vi "HDF5_Write_Disdrometer_Record.vi"(0 "DisdromRefs":T4 {"Status_dset_deprecated" format="%.0x"; "Spectrum_dset" format="%.0x"; "SpectGroup_ref" format="%.0x"; "HydromType_dset" format="%.0x"; "UnknownVolum_dset" format="%.0x"; "UnknownParticls_dset" format="%.0x"; "NonHydrVolum_dset" format="%.0x"; "NonHydrParticls_dset" format="%.0x"; "ParticlMinDiam_dset" format="%.0x"; "ParticlMaxSpeed_dset" format="%.0x"; "RadarReflect_dset" format="%.0x"; "Visibility_dset" format="%.0x"; "TotalRain_dset" format="%.0x"; "Solid_dset" format="%.0x"; "Liquid_dset" format="%.0x"; "TotalRainRate_dset" format="%.0x"; "TimeStamp_dset" format="%.0x"; "ParticlMinSpeed_dset" format="%.0x"; "MeasdParticles_dset" format="%.0x"; "MaxDiam_dset" format="%.0x"; "BasicGroup_ref" format="%.0x"}, 7 "DisdrometerData":T1={"Spectrum Data"=[], "DisdromSummary"={"current time"=0.0, "Timestamp"=0.0, "Total Rain Rate"=0.0, "Liquid Rain Rate"=0.0, "Solid Rain Rate"=0.0, "Total Rainfall"=0.0, "Visibility"=0.0, "Radar Reflectivity"=0.0, "Max Diameter Hail"=0.0, "Measured Particles"=0, "Particle Min Speed"=0, "Particle Max Speed"=0, "Particle Min Diam"=0, "NonHydr Particles"=0, "NonHydr Volume"=0.0, "Unkn Particles"=0, "Unkn Volume"=0.0, "HydroType"=0}, "Status"={"Laser"=TRUE, "Signal"=TRUE, "LaserTemp_Analog"=TRUE, "LaserTemp_Digital"=TRUE, "LaserCurrent_Analog"=TRUE, "LaserCurrent_Digital"=TRUE, "SensorSupply"=TRUE, "HeatLaserHead"=TRUE, "HeatReceiverHead"=TRUE, "TempSensor"=TRUE, "HeatSupply"=TRUE, "HeatHousing"=TRUE, "HeatHeads"=TRUE, "HeatCarriers"=TRUE, "OutputLaserPower"=TRUE, "Checksum"=TRUE, "StatusInt"=0}}, 11 "error in":errorcluster) -> (15 "error out":errorcluster)   [LabVIEW 2018]
doc: "Write a single Noise<x> record with timestamp:\nNoise1\n NoiseInfo - cluster with Timestamp and other metadata for this record\n SummdSpectrum - 1024 element Double array (waveform)"
uses:
  HDF5_Disdrometer_Refs.ctl
  <vilib>/addons/h5labview2/base/hid_t.ctl
  DisdrometerData.ctl
  DisdromterSummaryData.ctl
  Disdrometer/Disdrometer_Status_Cluster.ctl
  lib_path_mod_20200519.vi
  <vilib>/addons/h5labview2/base/H5Equery.vi
  <vilib>/addons/h5labview2/base/lib_path.vi
  <vilib>/addons/h5labview2/dataset/H5Dwrite.llb/H5Dwrite.xnode
  <vilib>/addons/h5labview2/dataset/H5D.lvlib
  <vilib>/addons/h5labview2/space/H5S.lvlib
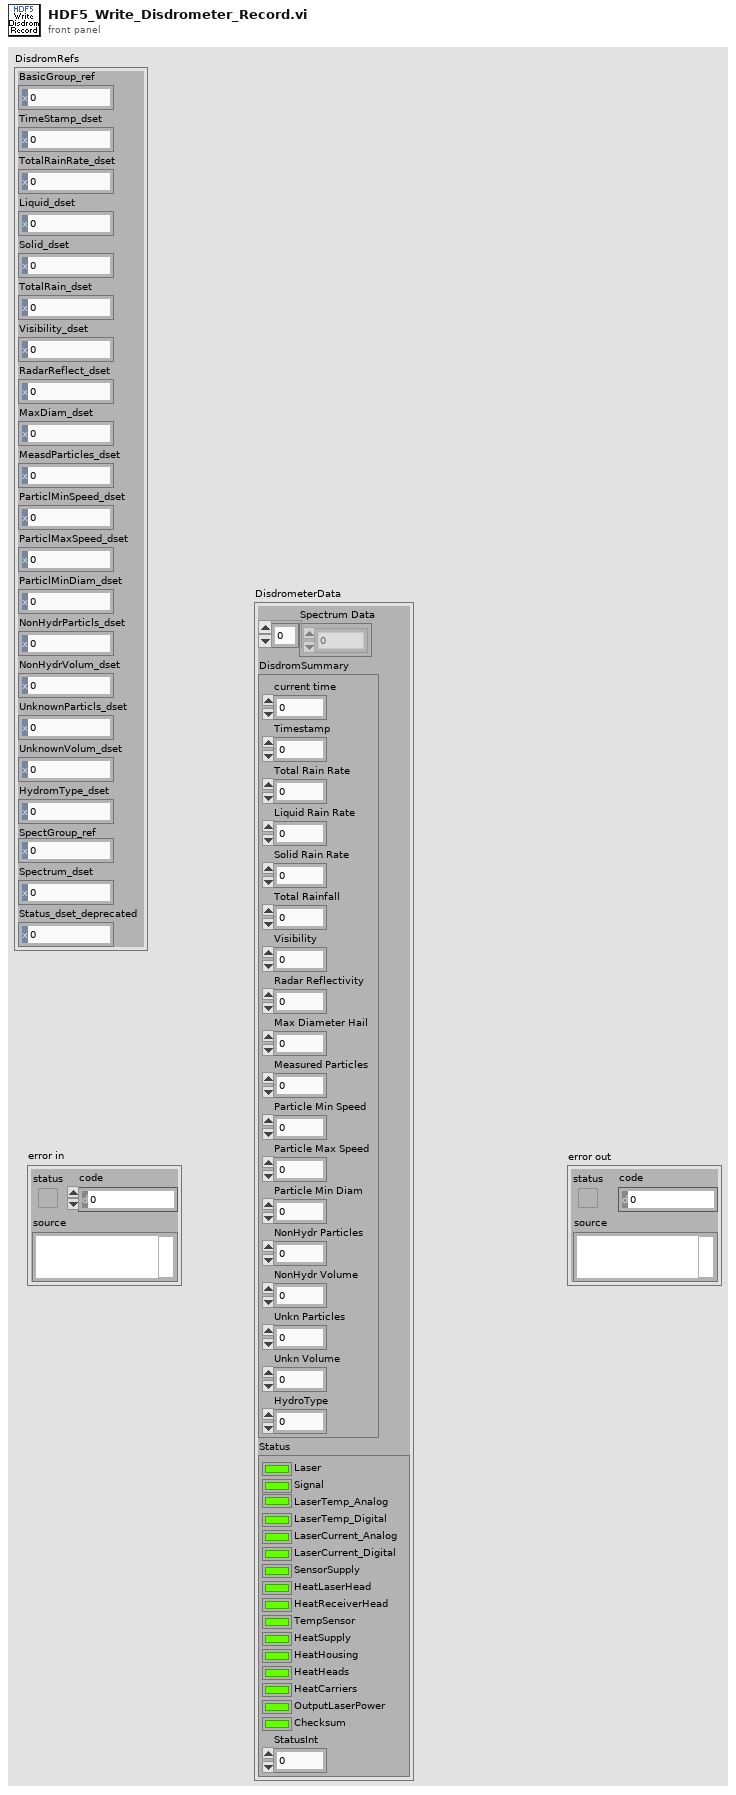
[diagram p1: front panel]
types:
  T1 = typedef "DisdrometerData.ctl" = cluster{"Spectrum Data":i16[], "DisdromSummary":T2, "Status":T3}
  T2 = typedef "DisdromterSummaryData.ctl" = cluster{"current time":dbl, "Timestamp":dbl, "Total Rain Rate":dbl, "Liquid Rain Rate":dbl, "Solid Rain Rate":dbl, "Total Rainfall":dbl, "Visibility":dbl, "Radar Reflectivity":dbl, "Max Diameter Hail":dbl, "Measured Particles":i32, "Particle Min Speed":i16, "Particle Max Speed":i16, "Particle Min Diam":i16, "NonHydr Particles":i16, "NonHydr Volume":dbl, "Unkn Particles":i16, "Unkn Volume":dbl, "HydroType":i8}
  T3 = typedef "Disdrometer_Status_Cluster.ctl" = cluster{"Laser":bool, "Signal":bool, "LaserTemp_Analog":bool, "LaserTemp_Digital":bool, "LaserCurrent_Analog":bool, "LaserCurrent_Digital":bool, "SensorSupply":bool, "HeatLaserHead":bool, "HeatReceiverHead":bool, "TempSensor":bool, "HeatSupply":bool, "HeatHousing":bool, "HeatHeads":bool, "HeatCarriers":bool, "OutputLaserPower":bool, "Checksum":bool, "StatusInt":u16}
  T4 = typedef "HDF5_Disdrometer_Refs.ctl" = cluster{"BasicGroup_ref":T5, "TimeStamp_dset":T5, "TotalRainRate_dset":T5, "Liquid_dset":T5, "Solid_dset":T5, "TotalRain_dset":T5, "Visibility_dset":T5, "RadarReflect_dset":T5, "MaxDiam_dset":T5, "MeasdParticles_dset":T5, "ParticlMinSpeed_dset":T5, "ParticlMaxSpeed_dset":T5, "ParticlMinDiam_dset":T5, "NonHydrParticls_dset":T5, "NonHydrVolum_dset":T5, "UnknownParticls_dset":T5, "UnknownVolum_dset":T5, "HydromType_dset":T5, "SpectGroup_ref":T5, "Spectrum_dset":T5, "Status_dset_deprecated":T5}
  T5 = typedef "hid_t.ctl" = i32
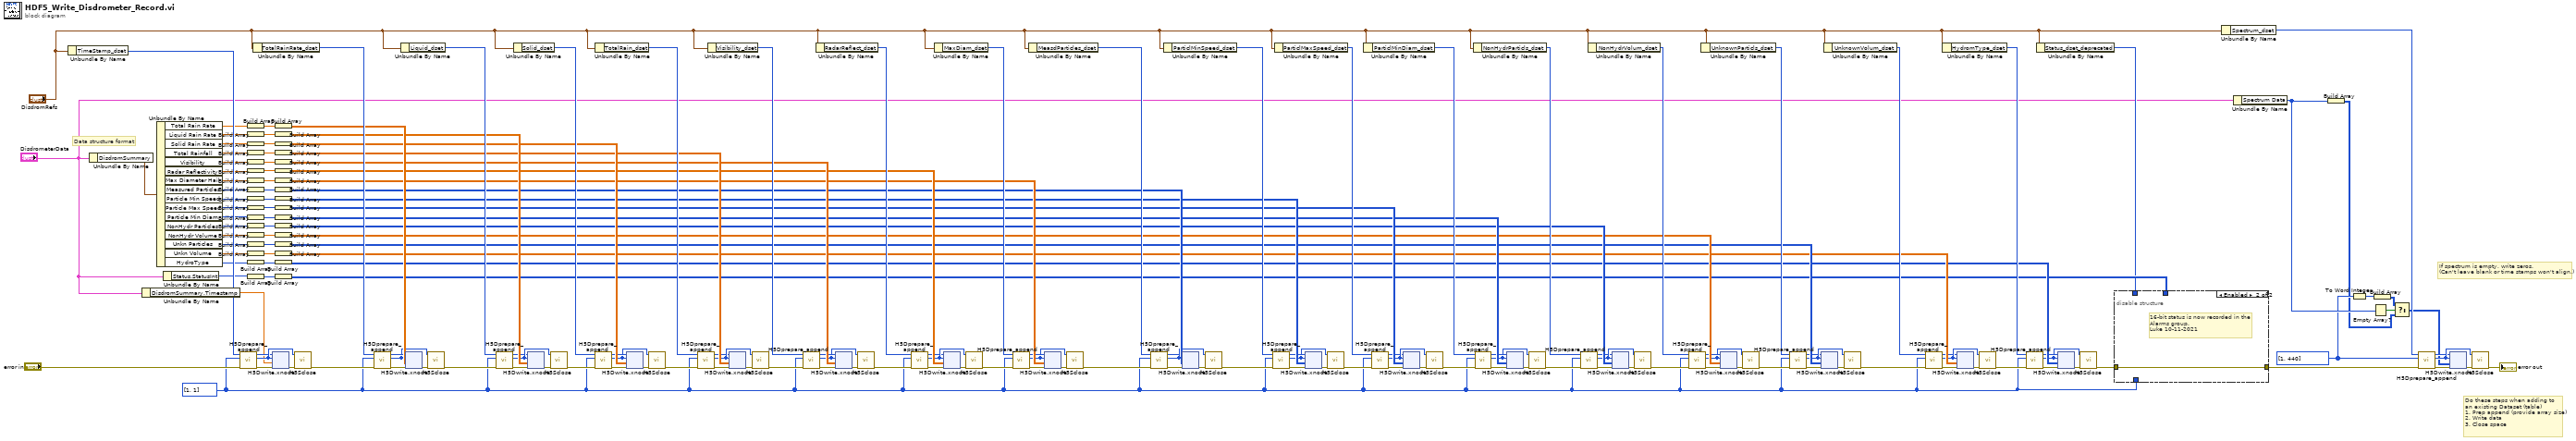
[diagram p0: block diagram]
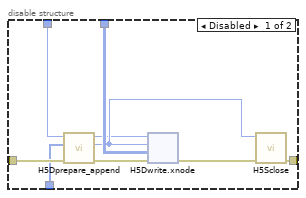
[diagram p2: hidden frame]
diagram:
  w6 = u64[] [1, 440] ("append dims")
  w17 = i32[] [1, 1] ("size(s)")
  # "If spectrum is empty, write zeros.\n(Can't leave blank or time stamps won't align.)"
  # "Data structure format"
  # "Do these steps when adding to \nan existing Dataset (table)\n1. Prep append (provide array size)\n2. Write data\n3. Close space"
  n1 = Unbundle By Name("DisdromRefs") -> ("TimeStamp_dset"=w174:T5)
  n2 = Unbundle By Name("DisdrometerData") -> ("DisdromSummary"=w132:T2)
  n3 = Unbundle By Name("DisdrometerData") -> ("DisdromSummary.Timestamp"=w1:dbl)
  n4 = Unbundle By Name(w132) -> ("Total Rain Rate"=w99:dbl, "Liquid Rain Rate"=w22:dbl, "Solid Rain Rate"=w23:dbl, "Total Rainfall"=w24:dbl, "Visibility"=w25:dbl, "Radar Reflectivity"=w26:dbl, "Max Diameter Hail"=w27:dbl, "Measured Particles"=w28:i32, "Particle Min Speed"=w29:i16, "Particle Max Speed"=w30:i16, "Particle Min Diam"=w31:i16, "NonHydr Particles"=w32:i16, "NonHydr Volume"=w33:dbl, "Unkn Particles"=w34:i16, "Unkn Volume"=w35:dbl, "HydroType"=w36:i8)
  n5 = Unbundle By Name("DisdrometerData") -> ("Status.StatusInt"=w21:u16)
  n6 = call <vilib>:"H5Dprepare_append.vi"("error in (no error)"="error in", "append dims"=w17, "dset in"=w174) -> ("error out"=w136:errorcluster, "space out"=w134:T5, "dset out"=w133:T5)  [unwired: 5 in, 1 out]
  n7 = Build Array(w99) -> (w52:dbl[])
  n8 = Build Array(w22) -> (w51:dbl[])
  n9 = Build Array(w23) -> (w49:dbl[])
  n10 = Build Array(w24) -> (w50:dbl[])
  n11 = Build Array(w25) -> (w45:dbl[])
  n12 = Build Array(w26) -> (w46:dbl[])
  n13 = Build Array(w27) -> (w48:dbl[])
  n14 = Build Array(w28) -> (w47:i32[])
  n15 = Build Array(w29) -> (w37:i16[])
  n16 = Build Array(w30) -> (w38:i16[])
  n17 = Build Array(w31) -> (w40:i16[])
  n18 = Build Array(w32) -> (w39:i16[])
  n19 = Build Array(w33) -> (w44:dbl[])
  n20 = Build Array(w34) -> (w43:i16[])
  n21 = Build Array(w35) -> (w41:dbl[])
  n22 = Build Array(w36) -> (w42:i8[])
  n23 = Build Array(w21) -> (w20:u16[])
  n24 = Unbundle By Name("DisdromRefs") -> ("TotalRainRate_dset"=w172:T5)
  n25 = xnode "H5Dwrite.xnode"("error in (no error)"=w136, "data"=w1, "file space"=w134, "ref in"=w133) -> ("error out"=w135:errorcluster)  [unwired: 3 in, 2 out]
  n26 = Build Array(w52) -> (w156:dbl[][])
  n27 = Build Array(w51) -> (w155:dbl[][])
  n28 = Build Array(w49) -> (w154:dbl[][])
  n29 = Build Array(w50) -> (w153:dbl[][])
  n30 = Build Array(w45) -> (w152:dbl[][])
  n31 = Build Array(w46) -> (w151:dbl[][])
  n32 = Build Array(w48) -> (w150:dbl[][])
  n33 = Build Array(w47) -> (w149:i32[][])
  n34 = Build Array(w37) -> (w148:i16[][])
  n35 = Build Array(w38) -> (w147:i16[][])
  n36 = Build Array(w40) -> (w146:i16[][])
  n37 = Build Array(w39) -> (w145:i16[][])
  n38 = Build Array(w44) -> (w144:dbl[][])
  n39 = Build Array(w43) -> (w143:i16[][])
  n40 = Build Array(w41) -> (w142:dbl[][])
  n41 = Build Array(w42) -> (w141:i8[][])
  n42 = Build Array(w20) -> (w16:u16[][])
  n43 = call <vilib>:"H5Sclose.vi"("error in (no error)"=w135, "space in"=w134) -> ("error out"=w118:errorcluster)  [unwired: 9 in]
  n44 = call <vilib>:"H5Dprepare_append.vi"("error in (no error)"=w118, "append dims"=w17, "dset in"=w172) -> ("error out"=w137:errorcluster, "space out"=w139:T5, "dset out"=w140:T5)  [unwired: 5 in, 1 out]
  n45 = Unbundle By Name("DisdromRefs") -> ("Liquid_dset"=w171:T5)
  n46 = xnode "H5Dwrite.xnode"("error in (no error)"=w137, "data"=w156, "file space"=w139, "ref in"=w140) -> ("error out"=w138:errorcluster)  [unwired: 3 in, 2 out]
  n47 = call <vilib>:"H5Sclose.vi"("error in (no error)"=w138, "space in"=w139) -> ("error out"=w117:errorcluster)  [unwired: 9 in]
  n48 = call <vilib>:"H5Dprepare_append.vi"("error in (no error)"=w117, "append dims"=w17, "dset in"=w171) -> ("error out"=w131:errorcluster, "space out"=w129:T5, "dset out"=w128:T5)  [unwired: 5 in, 1 out]
  n49 = Unbundle By Name("DisdromRefs") -> ("Solid_dset"=w170:T5)
  n50 = xnode "H5Dwrite.xnode"("error in (no error)"=w131, "data"=w155, "file space"=w129, "ref in"=w128) -> ("error out"=w130:errorcluster)  [unwired: 3 in, 2 out]
  n51 = call <vilib>:"H5Sclose.vi"("error in (no error)"=w130, "space in"=w129) -> ("error out"=w116:errorcluster)  [unwired: 9 in]
  n52 = call <vilib>:"H5Dprepare_append.vi"("error in (no error)"=w116, "append dims"=w17, "dset in"=w170) -> ("error out"=w124:errorcluster, "space out"=w126:T5, "dset out"=w127:T5)  [unwired: 5 in, 1 out]
  n53 = Unbundle By Name("DisdromRefs") -> ("TotalRain_dset"=w169:T5)
  n54 = xnode "H5Dwrite.xnode"("error in (no error)"=w124, "data"=w154, "file space"=w126, "ref in"=w127) -> ("error out"=w125:errorcluster)  [unwired: 3 in, 2 out]
  n55 = call <vilib>:"H5Sclose.vi"("error in (no error)"=w125, "space in"=w126) -> ("error out"=w115:errorcluster)  [unwired: 9 in]
  n56 = call <vilib>:"H5Dprepare_append.vi"("error in (no error)"=w115, "append dims"=w17, "dset in"=w169) -> ("error out"=w123:errorcluster, "space out"=w121:T5, "dset out"=w120:T5)  [unwired: 5 in, 1 out]
  n57 = Unbundle By Name("DisdromRefs") -> ("Visibility_dset"=w168:T5)
  n58 = xnode "H5Dwrite.xnode"("error in (no error)"=w123, "data"=w153, "file space"=w121, "ref in"=w120) -> ("error out"=w122:errorcluster)  [unwired: 3 in, 2 out]
  n59 = call <vilib>:"H5Sclose.vi"("error in (no error)"=w122, "space in"=w121) -> ("error out"=w110:errorcluster)  [unwired: 9 in]
  n60 = call <vilib>:"H5Dprepare_append.vi"("error in (no error)"=w110, "append dims"=w17, "dset in"=w168) -> ("error out"=w111:errorcluster, "space out"=w113:T5, "dset out"=w114:T5)  [unwired: 5 in, 1 out]
  n61 = Unbundle By Name("DisdromRefs") -> ("RadarReflect_dset"=w167:T5)
  n62 = xnode "H5Dwrite.xnode"("error in (no error)"=w111, "data"=w152, "file space"=w113, "ref in"=w114) -> ("error out"=w112:errorcluster)  [unwired: 3 in, 2 out]
  n63 = call <vilib>:"H5Sclose.vi"("error in (no error)"=w112, "space in"=w113) -> ("error out"=w105:errorcluster)  [unwired: 9 in]
  n64 = call <vilib>:"H5Dprepare_append.vi"("error in (no error)"=w105, "append dims"=w17, "dset in"=w167) -> ("error out"=w109:errorcluster, "space out"=w107:T5, "dset out"=w106:T5)  [unwired: 5 in, 1 out]
  n65 = Unbundle By Name("DisdromRefs") -> ("MaxDiam_dset"=w166:T5)
  n66 = xnode "H5Dwrite.xnode"("error in (no error)"=w109, "data"=w151, "file space"=w107, "ref in"=w106) -> ("error out"=w108:errorcluster)  [unwired: 3 in, 2 out]
  n67 = call <vilib>:"H5Sclose.vi"("error in (no error)"=w108, "space in"=w107) -> ("error out"=w100:errorcluster)  [unwired: 9 in]
  n68 = call <vilib>:"H5Dprepare_append.vi"("error in (no error)"=w100, "append dims"=w17, "dset in"=w166) -> ("error out"=w101:errorcluster, "space out"=w103:T5, "dset out"=w104:T5)  [unwired: 5 in, 1 out]
  n69 = Unbundle By Name("DisdromRefs") -> ("MeasdParticles_dset"=w159:T5)
  n70 = xnode "H5Dwrite.xnode"("error in (no error)"=w101, "data"=w150, "file space"=w103, "ref in"=w104) -> ("error out"=w102:errorcluster)  [unwired: 3 in, 2 out]
  n71 = call <vilib>:"H5Sclose.vi"("error in (no error)"=w102, "space in"=w103) -> ("error out"=w64:errorcluster)  [unwired: 9 in]
  n72 = call <vilib>:"H5Dprepare_append.vi"("error in (no error)"=w64, "append dims"=w17, "dset in"=w159) -> ("error out"=w68:errorcluster, "space out"=w66:T5, "dset out"=w65:T5)  [unwired: 5 in, 1 out]
  n73 = Unbundle By Name("DisdromRefs") -> ("ParticlMinSpeed_dset"=w160:T5)
  n74 = xnode "H5Dwrite.xnode"("error in (no error)"=w68, "data"=w149, "file space"=w66, "ref in"=w65) -> ("error out"=w67:errorcluster)  [unwired: 3 in, 2 out]
  n75 = call <vilib>:"H5Sclose.vi"("error in (no error)"=w67, "space in"=w66) -> ("error out"=w81:errorcluster)  [unwired: 9 in]
  n76 = call <vilib>:"H5Dprepare_append.vi"("error in (no error)"=w81, "append dims"=w17, "dset in"=w160) -> ("error out"=w69:errorcluster, "space out"=w71:T5, "dset out"=w72:T5)  [unwired: 5 in, 1 out]
  n77 = Unbundle By Name("DisdromRefs") -> ("ParticlMaxSpeed_dset"=w161:T5)
  n78 = xnode "H5Dwrite.xnode"("error in (no error)"=w69, "data"=w148, "file space"=w71, "ref in"=w72) -> ("error out"=w70:errorcluster)  [unwired: 3 in, 2 out]
  n79 = call <vilib>:"H5Sclose.vi"("error in (no error)"=w70, "space in"=w71) -> ("error out"=w82:errorcluster)  [unwired: 9 in]
  n80 = Unbundle By Name("DisdromRefs") -> ("ParticlMinDiam_dset"=w162:T5)
  n81 = call <vilib>:"H5Dprepare_append.vi"("error in (no error)"=w82, "append dims"=w17, "dset in"=w161) -> ("error out"=w76:errorcluster, "space out"=w74:T5, "dset out"=w73:T5)  [unwired: 5 in, 1 out]
  n82 = xnode "H5Dwrite.xnode"("error in (no error)"=w76, "data"=w147, "file space"=w74, "ref in"=w73) -> ("error out"=w75:errorcluster)  [unwired: 3 in, 2 out]
  n83 = call <vilib>:"H5Sclose.vi"("error in (no error)"=w75, "space in"=w74) -> ("error out"=w83:errorcluster)  [unwired: 9 in]
  n84 = Unbundle By Name("DisdromRefs") -> ("NonHydrParticls_dset"=w163:T5)
  n85 = call <vilib>:"H5Dprepare_append.vi"("error in (no error)"=w83, "append dims"=w17, "dset in"=w162) -> ("error out"=w77:errorcluster, "space out"=w79:T5, "dset out"=w80:T5)  [unwired: 5 in, 1 out]
  n86 = xnode "H5Dwrite.xnode"("error in (no error)"=w77, "data"=w146, "file space"=w79, "ref in"=w80) -> ("error out"=w78:errorcluster)  [unwired: 3 in, 2 out]
  n87 = call <vilib>:"H5Sclose.vi"("error in (no error)"=w78, "space in"=w79) -> ("error out"=w88:errorcluster)  [unwired: 9 in]
  n88 = call <vilib>:"H5Dprepare_append.vi"("error in (no error)"=w88, "append dims"=w17, "dset in"=w163) -> ("error out"=w87:errorcluster, "space out"=w85:T5, "dset out"=w84:T5)  [unwired: 5 in, 1 out]
  n89 = Unbundle By Name("DisdromRefs") -> ("NonHydrVolum_dset"=w164:T5)
  n90 = xnode "H5Dwrite.xnode"("error in (no error)"=w87, "data"=w145, "file space"=w85, "ref in"=w84) -> ("error out"=w86:errorcluster)  [unwired: 3 in, 2 out]
  n91 = call <vilib>:"H5Sclose.vi"("error in (no error)"=w86, "space in"=w85) -> ("error out"=w93:errorcluster)  [unwired: 9 in]
  n92 = call <vilib>:"H5Dprepare_append.vi"("error in (no error)"=w93, "append dims"=w17, "dset in"=w164) -> ("error out"=w89:errorcluster, "space out"=w91:T5, "dset out"=w92:T5)  [unwired: 5 in, 1 out]
  n93 = Unbundle By Name("DisdromRefs") -> ("UnknownParticls_dset"=w165:T5)
  n94 = xnode "H5Dwrite.xnode"("error in (no error)"=w89, "data"=w144, "file space"=w91, "ref in"=w92) -> ("error out"=w90:errorcluster)  [unwired: 3 in, 2 out]
  n95 = call <vilib>:"H5Sclose.vi"("error in (no error)"=w90, "space in"=w91) -> ("error out"=w98:errorcluster)  [unwired: 9 in]
  n96 = call <vilib>:"H5Dprepare_append.vi"("error in (no error)"=w98, "append dims"=w17, "dset in"=w165) -> ("error out"=w97:errorcluster, "space out"=w95:T5, "dset out"=w94:T5)  [unwired: 5 in, 1 out]
  n97 = xnode "H5Dwrite.xnode"("error in (no error)"=w97, "data"=w143, "file space"=w95, "ref in"=w94) -> ("error out"=w96:errorcluster)  [unwired: 3 in, 2 out]
  n98 = Unbundle By Name("DisdromRefs") -> ("UnknownVolum_dset"=w158:T5)
  n99 = call <vilib>:"H5Sclose.vi"("error in (no error)"=w96, "space in"=w95) -> ("error out"=w54:errorcluster)  [unwired: 9 in]
  n100 = call <vilib>:"H5Dprepare_append.vi"("error in (no error)"=w54, "append dims"=w17, "dset in"=w158) -> ("error out"=w63:errorcluster, "space out"=w61:T5, "dset out"=w60:T5)  [unwired: 5 in, 1 out]
  n101 = Unbundle By Name("DisdromRefs") -> ("HydromType_dset"=w157:T5)
  n102 = xnode "H5Dwrite.xnode"("error in (no error)"=w63, "data"=w142, "file space"=w61, "ref in"=w60) -> ("error out"=w62:errorcluster)  [unwired: 3 in, 2 out]
  n103 = call <vilib>:"H5Sclose.vi"("error in (no error)"=w62, "space in"=w61) -> ("error out"=w55:errorcluster)  [unwired: 9 in]
  n104 = call <vilib>:"H5Dprepare_append.vi"("error in (no error)"=w55, "append dims"=w17, "dset in"=w157) -> ("error out"=w56:errorcluster, "space out"=w58:T5, "dset out"=w59:T5)  [unwired: 5 in, 1 out]
  n105 = Unbundle By Name("DisdromRefs") -> ("Status_dset_deprecated"=w14:T5)
  n106 = xnode "H5Dwrite.xnode"("error in (no error)"=w56, "data"=w141, "file space"=w58, "ref in"=w59) -> ("error out"=w57:errorcluster)  [unwired: 3 in, 2 out]
  n107 = call <vilib>:"H5Sclose.vi"("error in (no error)"=w57, "space in"=w58) -> ("error out"=w19:errorcluster)  [unwired: 9 in]
  n108 = disable-structure shown="Enabled" {
    disable-tunnel: w19 -> [w181 w203]
    disable-tunnel: [w180 w203] -> w18
    disable-tunnel: w17 -> [w179 _]
    disable-tunnel: w16 -> [w178 _]
    disable-tunnel: w14 -> [w175 _]
    frame Disabled {
      n109 = call <vilib>:"H5Dprepare_append.vi"("error in (no error)"=w181, "append dims"=w179, "dset in"=w175) -> ("error out"=w183:errorcluster, "space out"=w177:T5, "dset out"=w176:T5)  [unwired: 5 in, 1 out]
      n110 = xnode "H5Dwrite.xnode"("error in (no error)"=w183, "data"=w178, "file space"=w177, "ref in"=w176) -> ("error out"=w182:errorcluster)  [unwired: 3 in, 2 out]
      n111 = call <vilib>:"H5Sclose.vi"("error in (no error)"=w182, "space in"=w177) -> ("error out"=w180:errorcluster)  [unwired: 9 in]
    }
    frame Enabled {
      # "16-bit status is now recorded in the \nAlarms group.\nLuke 10-11-2021"
    }
  }
  n112 = Unbundle By Name("DisdromRefs") -> ("Spectrum_dset"=w173:T5)
  n113 = Unbundle By Name("DisdrometerData") -> ("Spectrum Data"=w13:i16[])
  n114 = Build Array(w13) -> (w5:i16[][])
  n115 = To Word Integer(number=w6) -> (16bit integer=w3:i16[])
  n116 = Empty Array?(array=w13) -> (empty?=w8:bool)
  n117 = Build Array(w3) -> (w7:i16[][])
  n118 = Select(t=w7, s=w8, f=w5) -> (s? t:f=w4:i16[][])
  n119 = call <vilib>:"H5Dprepare_append.vi"("error in (no error)"=w18, "append dims"=w6, "dset in"=w173) -> ("error out"=w12:errorcluster, "space out"=w10:T5, "dset out"=w9:T5)  [unwired: 5 in, 1 out]
  n120 = xnode "H5Dwrite.xnode"("error in (no error)"=w12, "data"=w4, "file space"=w10, "ref in"=w9) -> ("error out"=w11:errorcluster)  [unwired: 3 in, 2 out]
  n121 = call <vilib>:"H5Sclose.vi"("error in (no error)"=w11, "space in"=w10) -> ("error out"=→"error out":errorcluster)  [unwired: 9 in]
